vi "Get Cache Params.vi"(8 "error in (no error)":errorcluster, 11 "Response in":refnum<class "Response.lvclass">) -> (0 "error out":errorcluster, 2 "Cache Params":T1={"Enabled"=FALSE, "Directive"=enum."None (no-store)", "Max Age"=0, "Immutable"=FALSE, "Last Modified"=timestamp(0 s since 1904-01-01), "Expires"=timestamp(0 s since 1904-01-01), "ETag"="", "Weak ETag"=FALSE}, 3 "Response out":refnum<class "Response.lvclass">)   [LabVIEW 2020, in "HTTP Utils.lvlib" / "Response.lvclass"]
uses:
  Response.lvclass
  Cache Directive.ctl
  HTTP Utils.lvlib
  Cache Params.ctl
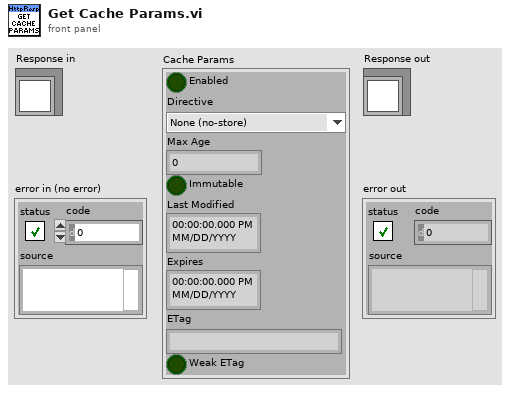
[diagram p1: front panel]
types:
  T1 = typedef "HTTP Utils.lvlib/Cache Params.ctl" = cluster{"Enabled":bool, "Directive":T2, "Max Age":i32, "Immutable":bool, "Last Modified":timestamp, "Expires":timestamp, "ETag":string, "Weak ETag":bool}
  T2 = typedef "HTTP Utils.lvlib/Cache Directive.ctl" = enum16{"Not Specified", "None (no-store)", "Always Validate (no-cache)", "Private Only (private)", "Always Allow (public)"}
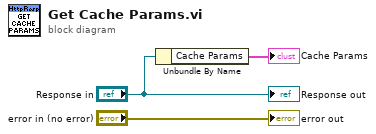
[diagram p0: block diagram]
diagram:
  n1 = Unbundle By Name("Response in") -> ("Cache Params"=→"Cache Params":T1)
  "error out" <- "error in (no error)"
  "Response out" <- "Response in"
